vi "Wiimote Parse Basic IR Point.vi"(0 "Byte 0 in":u8, 5 "Byte 1 in":u8, 7 "Byte 2 in":u8, 9 "Byte 3 in":u8, 11 "Byte 4 in":u8) -> (4 "Wiimote Point 1 out":T1, 15 "Wiimote Point 2 out":T1)   [LabVIEW 2011, in "Wiimote.lvlib"]
uses:
  Wiimote.lvlib
  Wiimote Point.ctl
panel:
  in  "Wiimote Point":T1
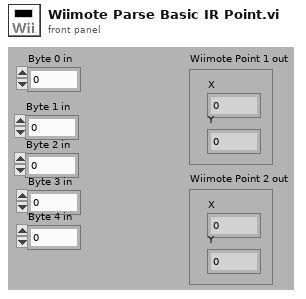
[diagram p1: front panel]
types:
  T1 = typedef "Wiimote.lvlib/Wiimote Point.ctl" = cluster{"X":u16, "Y":u16}
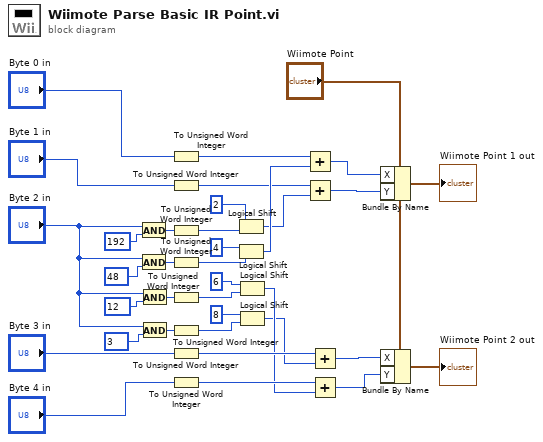
[diagram p0: block diagram]
diagram:
  n1 = And(x="Byte 2 in", y=u8 192 ("index")) -> (x .and. y?=w32:u8)
  n2 = And(x="Byte 2 in", y=u8 48 ("index")) -> (x .and. y?=w31:u8)
  n3 = And(x="Byte 2 in", y=u8 12 ("index")) -> (x .and. y?=w30:u8)
  n4 = And(x="Byte 2 in", y=u8 3 ("index")) -> (x .and. y?=w29:u8)
  n5 = To Unsigned Word Integer(number="Byte 0 in") -> (unsigned 16bit integer=w20:u16)
  n6 = To Unsigned Word Integer(number="Byte 1 in") -> (unsigned 16bit integer=w17:u16)
  n7 = To Unsigned Word Integer(number=w32) -> (unsigned 16bit integer=w28:u16)
  n8 = To Unsigned Word Integer(number=w31) -> (unsigned 16bit integer=w27:u16)
  n9 = To Unsigned Word Integer(number=w30) -> (unsigned 16bit integer=w26:u16)
  n10 = To Unsigned Word Integer(number=w29) -> (unsigned 16bit integer=w25:u16)
  n11 = To Unsigned Word Integer(number="Byte 3 in") -> (unsigned 16bit integer=w15:u16)
  n12 = To Unsigned Word Integer(number="Byte 4 in") -> (unsigned 16bit integer=w16:u16)
  n13 = Logical Shift(y=u16 2, x=w28) -> (x << y=w18:u16)
  n14 = Logical Shift(y=u16 4, x=w27) -> (x << y=w19:u16)
  n15 = Logical Shift(y=u16 6, x=w26) -> (x << y=w14:u16)
  n16 = Logical Shift(y=u16 8, x=w25) -> (x << y=w13:u16)
  n17 = Add(x=w20, y=w19) -> (x+y=w8:u16)
  n18 = Add(x=w17, y=w18) -> (x+y=w7:u16)
  n19 = Add(x=w15, y=w13) -> (x+y=w3:u16)
  n20 = Add(x=w16, y=w14) -> (x+y=w2:u16)
  n21 = Bundle By Name(cluster="Wiimote Point", "X"=w8, "Y"=w7) -> (→"Wiimote Point 1 out":T1)
  n22 = Bundle By Name(cluster="Wiimote Point", "X"=w3, "Y"=w2) -> (→"Wiimote Point 2 out":T1)
